vi "Update Fit Plot.vi"(8 "error in (no error)":errorcluster, 11 "Resonance Detector in":refnum<class "Resonance Detector.lvclass">) -> (0 "error out":errorcluster, 3 "Resonance Detector out":refnum<class "Resonance Detector.lvclass">)   [LabVIEW 2020, in "Resonance Detector.lvclass"]
uses:
  Resonance Detector.lvclass
  Resonance Detector.lvclass/Resonance Detector.ctl
  Read Line detector configuration.vi
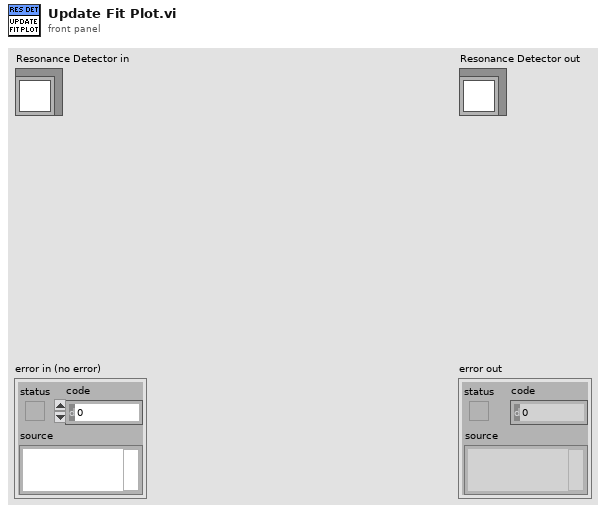
[diagram p1: front panel]
types:
  T1 = typedef "Line Detector Configuration.ctl" = cluster{"Peak width guess":dbl, "Background removal":enum16{"NONE", "High-pass", "Detrend"}, "Smoothing":enum16{"NONE", "Low-pass", "Denoise"}, "Smooth window":dbl, "Relative threshold":dbl, "Finder algorithm":enum16{"Basic", "Wavelet", "Wavelet+detrend"}, "Bgd window":dbl, "Spectrum recorder module name":string, "Fit window":dbl, "Initial fit guess":enum16{"Peak finder", "Last fit"}, "Follow\npeaks":bool, "Re-sample":dbl}
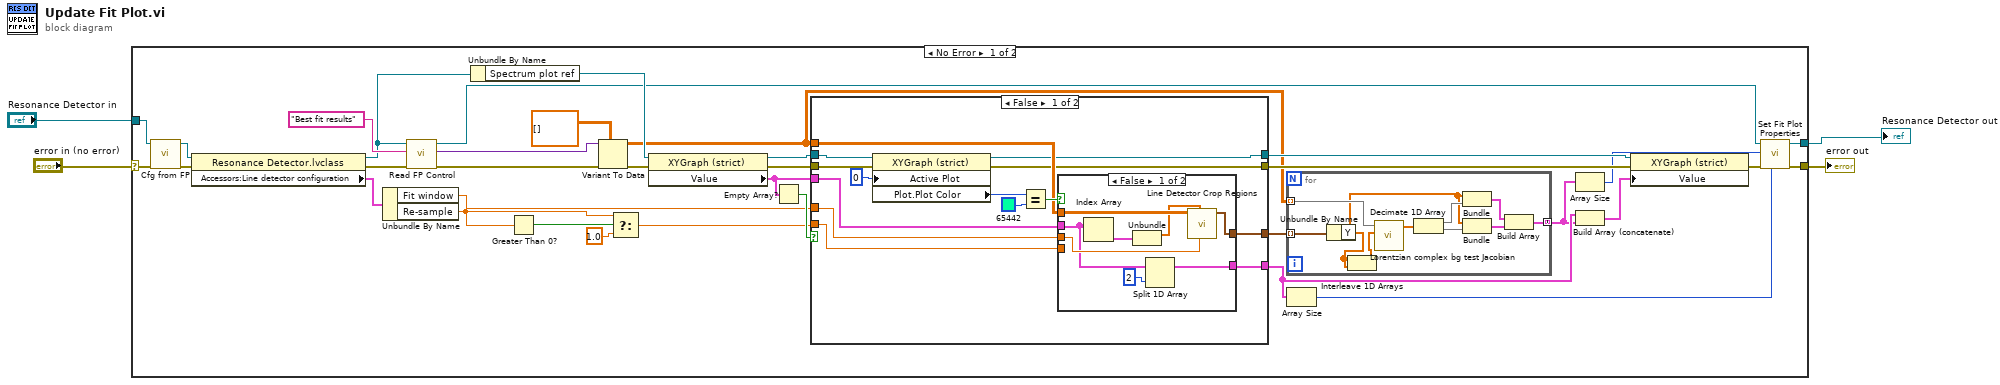
[diagram p0: block diagram]
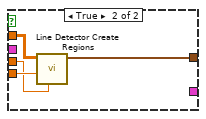
[diagram p2: hidden frame]
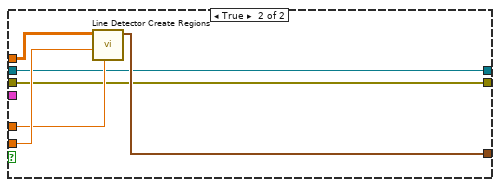
[diagram p3: hidden frame]
diagram:
  n1 = case shown="No Error" "error in (no error)" {
    selector: "error in (no error)" -> [w22 w83]
    tunnel: [w18 w83] -> w3
    tunnel: [w24 w82] -> w1
    tunnel: "Resonance Detector in" -> [w37 w82]
    frame No Error {
      n2 = call-dynamic "Cfg from FP.vi"("error in (no error)"=w22, "Measure Object in"=w37) -> ("error out"=w36:errorcluster, "Measure Object out"=w25:refnum<class "Resonance Detector.lvclass">)  [unwired: 8 in]
      n3 = property class="Resonance Detector.lvclass"(reference=w25, error in=w36) -> (reference out=w8:refnum<class "Resonance Detector.lvclass">, error out=w11:errorcluster, "Accessors:Line detector configuration"=w35:T1)
      n4 = Unbundle By Name(w35) -> ("Fit window"=w28:dbl, "Re-sample"=w33:dbl)
      n5 = call-dynamic "Read FP Control.vi"("error in (no error)"=w11, "Control Name"="Best fit results", "Measure Object in"=w8) -> ("error out"=w14:errorcluster, "Control Value"=w13:variant, "Measure Object out"=w9:refnum<class "Resonance Detector.lvclass">)  [unwired: 5 in, 1 out]
      n6 = Unbundle By Name(w8) -> ("Spectrum plot ref"=w39:refnum<vi>)
      n7 = Greater Than 0?(x=w33) -> (x > 0?=w34:bool)
      n8 = Variant To Data(error in=w14, type=dbl[][] [] ("Best fit results"), Variant=w13) -> (data=w7:dbl[][], error out=w10:errorcluster)
      n9 = Select(t=w33, s=w34, f=1.0) -> (s? t:f=w29:dbl)
      n10 = property class="XYGraph (strict)"(reference=w39, error in=w10) -> (reference out=w38:refnum<vi>, error out=w31:errorcluster, "Value"=w27:cluster{dbl[], dbl[]}[])
      n11 = Empty Array?(array=w27) -> (empty?=w30:bool)
      n12 = case shown="False" w30 {
        tunnel: w38 -> [w63 w76]
        tunnel: w31 -> [w62 w77]
        tunnel: w29 -> [w57 w80]
        tunnel: w7 -> [w56 w81]
        tunnel: w28 -> [w55 w79]
        tunnel: w27 -> [w54 _]
        tunnel: [w53 w78] -> w26
        tunnel: [w52 _] -> w17
        tunnel: [w51 w77] -> w21
        tunnel: [w50 w76] -> w23
        frame False {
          n13 = property class="XYGraph (strict)"(reference=w63, error in=w62, "Active Plot"=u32 0) -> (reference out=w50:refnum<vi>, error out=w51:errorcluster, "Plot.Plot Color"=w60:u32)
          n14 = Equal?(x=w60, y=u32 65442 ("Color Box")) -> (x = y?=w58:bool)
          n15 = case shown="False" w58 {
            tunnel: w57 -> [_ w75]
            tunnel: w56 -> [w71 w74]
            tunnel: w55 -> [w70 w73]
            tunnel: [w69 w72] -> w53
            tunnel: w54 -> [w65 _]
            tunnel: [w64 _] -> w52
            frame False {
              n16 = Index Array(array=w65) -> (element=w68:cluster{dbl[], dbl[]})  [unwired: 1 in]
              n17 = Unbundle(w68) -> (w67:dbl[])  [unwired: 1 out]
              n18 = Split 1D Array(array=w65, index=2) -> (first subarray=w64:cluster{dbl[], dbl[]}[])  [unwired: 1 out]
              n19 = call "Line Detector Crop Regions.vi"("Region width"=w70, "Frequency"=w67, "Best fit"=w71) -> ("Regions frequencies"=w69:waveform(dbl)[])  [unwired: 7 in, 1 out]
            }
            frame True {
              n20 = call "Line Detector Create Regions.vi"("Region width"=w73, "Re-sample"=w75, "Best fit"=w74) -> ("Regions frequencies"=w72:waveform(dbl)[])  [unwired: 8 in]
            }
          }
        }
        frame True {
          n21 = call "Line Detector Create Regions.vi"("Region width"=w79, "Re-sample"=w80, "Best fit"=w81) -> ("Regions frequencies"=w78:waveform(dbl)[])  [unwired: 8 in]
        }
      }
      n22 = for {
        tunnel: w26 -> [w48] mode=indexing
        tunnel: w7 -> [w49] mode=indexing
        tunnel: [w42] -> w6 mode=concatenating
        n23 = Unbundle By Name(w48) -> ("Y"=w41:dbl[])
        n24 = Interleave 1D Arrays(w41, w41) -> (w40:dbl[])
        n25 = call "Lorentzian complex bg test Jacobian.vi"("X"=w40, "a"=w49) -> ("f(X,a)"=w47:dbl[])  [unwired: 2 in, 2 out]
        n26 = Decimate 1D Array(w47) -> (w46:dbl[], w45:dbl[])
        n27 = Bundle("Y"=w41, w46) -> (w44:cluster{"Y":dbl[], dbl[]})  [unwired: 1 in]
        n28 = Bundle("Y"=w41, w45) -> (w43:cluster{"Y":dbl[], dbl[]})  [unwired: 1 in]
        n29 = Build Array(w44, w43) -> (w42:cluster{"Y":dbl[], dbl[]}[])
      }
      n30 = Array Size(array=w17) -> (size(s)=w16:i32)
      n31 = Array Size(array=w6) -> (size(s)=w5:i32)
      n32 = Build Array (concatenate)(w17, w6) -> (w19:cluster{"Y":dbl[], dbl[]}[])
      n33 = property class="XYGraph (strict)"(reference=w23, error in=w21, "Value"=w19) -> (error out=w20:errorcluster)  [unwired: 1 out]
      n34 = call-dynamic "Set Fit Plot Properties.vi"("Fit array start"=w16, "error in (no error)"=w20, "Fit array size"=w5, "Resonance Detector in"=w9) -> ("error out"=w18:errorcluster, "Resonance Detector out"=w24:refnum<class "Resonance Detector.lvclass">)  [unwired: 6 in]
    }
    frame Error {
    }
  }
  "error out" <- w3
  "Resonance Detector out" <- w1
